vi "HW_Set_FPS_on_device.vi"(0 "VISA in":refnum<visa-resource-name>, 1 "Desired FPS":T1=enum."Optimal", 2 "Sensor board size":string, 3 "Current FPS":i32, 4 "Force update (F)":bool, 5 "Error in (no error)":errorcluster) -> (14 "VISA out":refnum<visa-resource-name>, 15 "FPS set on device":i32, 16 "FPS requested":i32, 17 "Bytes written":u32, 18 "VISA reply":string, 19 "Error out":errorcluster)   [LabVIEW 2018, in "HW Interaction.lvlib"]
uses:
  SubVi's/Controls/CTL_Acquisition_speed_selector.ctl
  HW Interaction.lvlib
  Common_Resources.lvlib
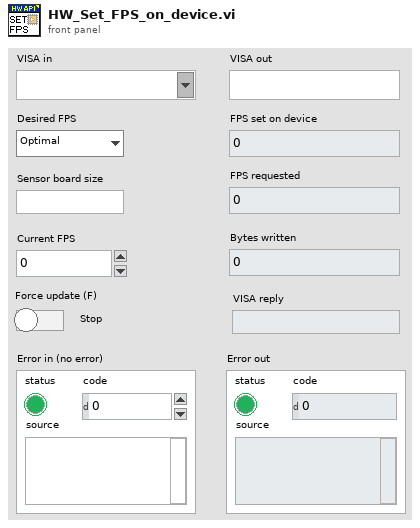
[diagram p1: front panel]
types:
  T1 = typedef "Common_Resources.lvlib/CTL_Acquisition_speed_selector.ctl" = enum16{"Max", "Optimal", "Eco"}
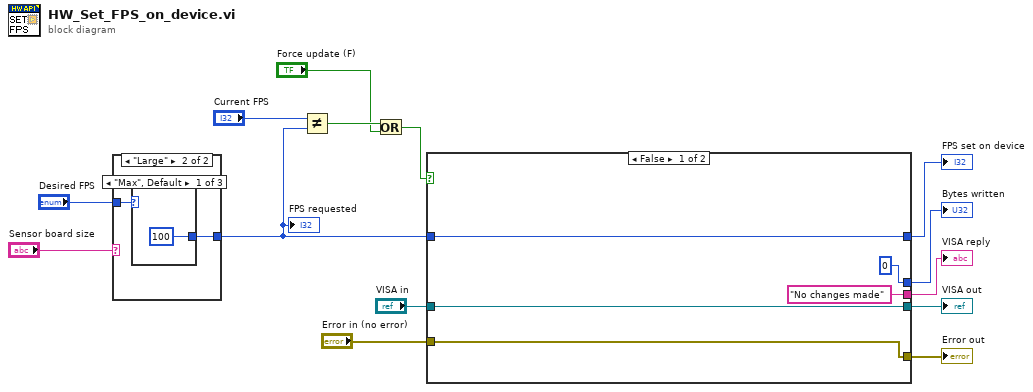
[diagram p0: block diagram]
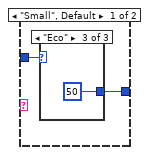
[diagram p2: hidden frame]
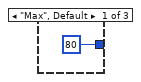
[diagram p3: hidden frame]
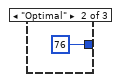
[diagram p4: hidden frame]
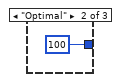
[diagram p5: hidden frame]
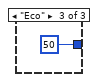
[diagram p6: hidden frame]
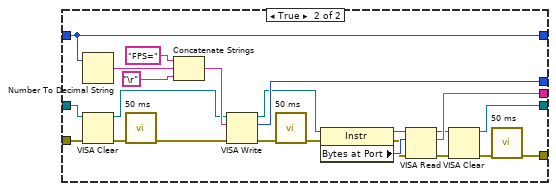
[diagram p7: hidden frame]
diagram:
  n1 = case shown="\"Large\"" "Sensor board size" {
    tunnel: "Desired FPS" -> [w16 w21]
    tunnel: [w15 w20] -> w12
    frame "Small", Default {
      n2 = case shown="\"Eco\"" w16 {
        tunnel: [80 76 50] -> w15
        frame "Max", Default {
        }
        frame "Optimal" {
        }
        frame "Eco" {
        }
      }
    }
    frame "Large" {
      n3 = case shown="\"Max\", Default" w21 {
        tunnel: [100 100 50] -> w20
        frame "Max", Default {
        }
        frame "Optimal" {
        }
        frame "Eco" {
        }
      }
    }
  }
  "FPS requested" <- w12
  n4 = Not Equal?(x="Current FPS", y=w12) -> (x != y?=w6:bool)
  n5 = Or(x=w6, y="Force update (F)") -> (x .or. y?=w5:bool)
  n6 = case shown="False" w5 {
    tunnel: "VISA in" -> [w29 w50]
    tunnel: "Error in (no error)" -> [w27 w45]
    tunnel: [w29 w31] -> w3
    tunnel: w12 -> [w28 w47]
    tunnel: [w28 w47] -> w8
    tunnel: [w27 w33] -> w9
    tunnel: [u32 0 ("return count") w41] -> w14
    tunnel: ["No changes made" ("read buffer") w35] -> w1
    frame False {
    }
    frame True {
      n7 = Number To Decimal String(number=w47) -> (decimal integer string=w48:string)  [unwired: 1 in]
      n8 = VISA Clear(VISA resource name=w50, error in (no error)=w45) -> (VISA resource name out=w46:refnum<visa-resource-name>, error out=w44:errorcluster)
      n9 = call "50 ms"("error in (no error)"=w44) -> ("error out"=w43:errorcluster)  [unwired: 10 in]
      n10 = Concatenate Strings("FPS=" ("write buffer"), w48, "\r") -> (w51:string)
      n11 = VISA Write(VISA resource name=w46, write buffer=w51, error in (no error)=w43) -> (VISA resource name out=w38:refnum<visa-resource-name>, return count=w41:u32, error out=w42:errorcluster)
      n12 = call "50 ms"("error in (no error)"=w42) -> ("error out"=w39:errorcluster)  [unwired: 10 in]
      n13 = property class="Instr"(reference=w38, error in=w39) -> (reference out=w36:refnum<visa-resource-name>, error out=w30:errorcluster, "Bytes at Port"=w37:u32)
      n14 = VISA Read(VISA resource name=w36, byte count=w37, error in (no error)=w30) -> (VISA resource name out=w32:refnum<visa-resource-name>, read buffer=w35:string, error out=w40:errorcluster)  [unwired: 1 out]
      n15 = VISA Clear(VISA resource name=w32, error in (no error)=w40) -> (VISA resource name out=w31:refnum<visa-resource-name>, error out=w34:errorcluster)
      n16 = call "50 ms"("error in (no error)"=w34) -> ("error out"=w33:errorcluster)  [unwired: 10 in]
    }
  }
  "Bytes written" <- w14
  "Error out" <- w9
  "FPS set on device" <- w8
  "VISA out" <- w3
  "VISA reply" <- w1
